vi "Locate Colored Object.vi"() -> ()   [LabVIEW 2013]
doc: "<B>Locate Colored Object</B> searches for objects of a color you select. There are three modes in this program. The first is \"Simple\" that lets you select red, green, or blue, and a sensitivity level. The second is \"Color Wheel\" which allows you to select a hue to search for along a color wheel. The final mode is \"HSL Numbers\" which allows you to set a minimum and maximum for Hue, Saturation, and Luminance. In all three cases a mask display shows any objects that match your parameters as red against a black background."
uses:
  <vilib>/Rock Robotics/WPI/Camera/WPI_CameraFrameRate.ctl
  <vilib>/Rock Robotics/WPI/Camera/WPI_CameraImageSize.ctl
panel:
  in  "Frame Rate (fps)":T1=20 min=1 max=30
  out "Mask":T2(plugin-control)
  out "Rectangle":T3
  in  "Tab Control":enum32{"Simple", "Color Wheel", "HSL Numbers"}(tab)=enum."Color Wheel"
  in  "Sensitivity":dbl(slide) scale=1.0..5.0
  in  "Basic Color":enum32{"Red", "Green", "Blue"}(radio)=enum."Green"
  in  "AutoCal":bool
  in  "Hue Selector":T4={"Hue"=65.11832883917573, "Saturation"=43.78787878787879, "Luminance"=100.45454545454545, "Hue Margin"=20.0} {"Hue Margin" scale=0.0..40.0; "Luminance" scale=0.0..255.0; "Saturation" scale=0.0..255.0; "Hue" scale=0.0..255.0}
  in  "Color Range":T5={"Hue"={"Lower"=55, "Upper"=93}, "Saturation"={"Lower"=73, "Upper"=255}, " Luminance"={"Lower"=99, "Upper"=255}}
  out "fps":dbl=20.0
  out "Particles":i32
  out "Area":i32
  in  "Decimate by":cluster{"H":i32, "V":i32}={"H"=3, "V"=5}
  in  "stop":bool
  # "This example shows a basic object location technique based on color processing.\nIt sets the camera up for medium sized image and passes each images into a subVI\nthat returns the location and size of the largest particle of that color. You can modify the\namount that you decimate the the image to trade speed for precision in location and size.\nThere are three ways to specify the color range.\nThe Simple tab implements a basic autoCalibration, Color wheel uses a center Hue and\nmargin amount, and a saturation and luminance range. The HSL numbers shows the low\nlevel values for complete flexibility."
  # "Determine which color best\ndescribes the target.\n\nMake sure it is in the frame\nand close to the camera,\nthen  press Calibrate.\n\nHigher Sensitivity tightens\nthe fit."
  # "Adjust the color"
  # "You can directly type in HSL threshold numbers.\nThis provides maximum control, but it helps to know\nwhat HSL is. Wikipedia may be able to help with that."
  # "Lower:"
  # "Upper:"
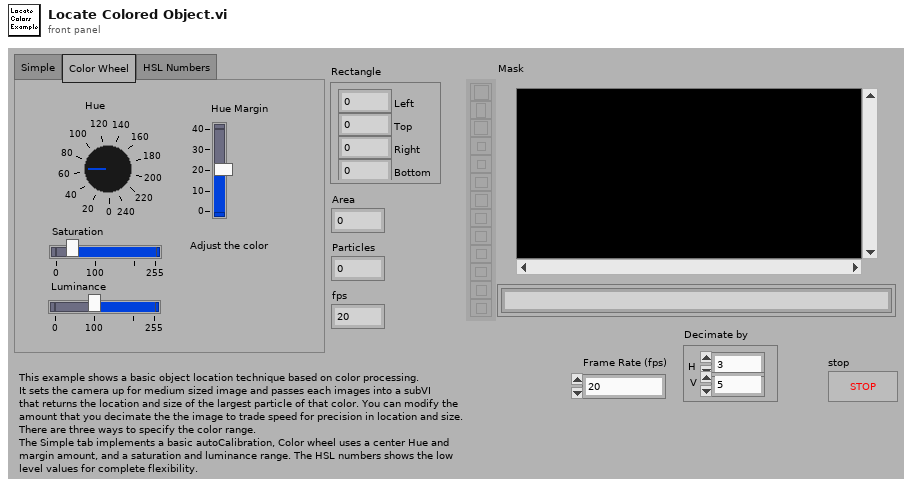
[diagram p1: front panel]
types:
  T1 = typedef "WPI_CameraFrameRate.ctl" = u32
  T2 = typedef "IMAQ Image.ctl" = refnum<image>
  T3 = cluster{"Left":i32, "Top":i32, "Right":i32, "Bottom":i32}
  T4 = cluster{"Hue":dbl, "Saturation":dbl, "Luminance":dbl, "Hue Margin":dbl}
  T5 = cluster{"Hue":cluster{"Lower":u8, "Upper":u8}, "Saturation":cluster{"Lower":u8, "Upper":u8}, " Luminance":cluster{"Lower":u8, "Upper":u8}}
  T6 = typedef "WPI_CameraImageSize.ctl" = enum16{"640x480", "320x240", "160x120"}
  T7 = typedef "Image Type" = u32
  T8 = typedef "WPI_CameraDevRef.ctl" = cluster{"Camera Address":string, "CameraStatus":errorcluster, "Acquire Image Notifier":refnum<notifier>}
  T9 = cluster{cluster{dbl, dbl}, cluster{"Saturation":dbl, i32}, cluster{"Luminance":dbl, i32}}
  T10 = cluster{cluster{sgl, sgl}, cluster{"Mean Value":sgl, "Standard  Deviation":sgl}}
  T11 = cluster{"Mean Value":sgl, "Standard  Deviation":sgl}
  T12 = cluster{cluster{sgl, sgl}, cluster{sgl, sgl}, cluster{sgl, sgl}}
  T13 = cluster{"Mean Value":sgl, sgl, sgl, "Standard  Deviation":sgl}
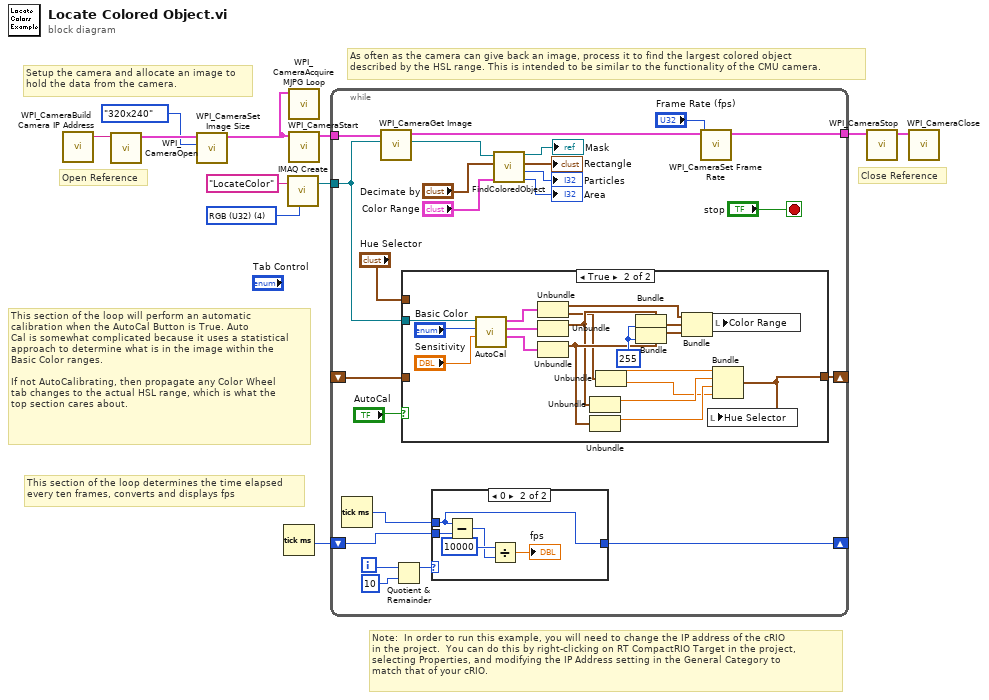
[diagram p0: block diagram]
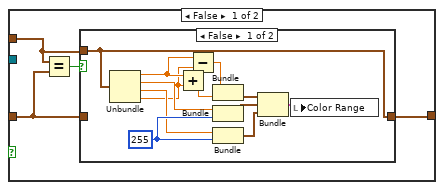
[diagram p2: hidden frame]
diagram:
  w6 = T7 4 items=["Grayscale (U8)", "Grayscale (I16)", "Grayscale (SGL)", "Complex (CSG)", "RGB (U32)", "HSL (U32)", "RGB (U64)", "Grayscale (U16)"] ("Image Type")
  # "Open Reference"
  # "Close Reference"
  # "Note:  In order to run this example, you will need to change the IP address of the cRIO\nin the project.  You can do this by right-clicking on RT CompactRIO Target in the project,\nselecting Properties, and modifying the IP Address setting in the General Category to \nmatch that of your cRIO."
  # "As often as the camera can give back an image, process it to find the largest colored object\ndescribed by the HSL range. This is intended to be similar to the functionality of the CMU camera."
  # "Setup the camera and allocate an image to\nhold the data from the camera."
  # "This section of the loop will perform an automatic\ncalibration when the AutoCal Button is True. Auto\nCal is somewhat complicated because it uses a statistical\napproach to determine what is in the image within the\nBasic Color ranges.\n\nIf not AutoCalibrating, then propagate any Color Wheel\ntab changes to the actual HSL range, which is what the\ntop section cares about."
  # "This section of the loop determines the time elapsed\nevery ten frames, converts and displays fps"
  n1 = call <vilib>:"WPI_CameraBuild Camera IP Address.vi"() -> ("Camera Address"=w2:string)  [unwired: 11 in]
  n2 = call <vilib>:"WPI_CameraOpen.vi"("Camera Address"=w2) -> ("CameraDevRef"=w4:T8)  [unwired: 1 in, 9 out]
  n3 = call <vilib>:"WPI_CameraSet Image Size.vi"("Image Size"=WPI_CameraImageSize."320x240", "CameraDevRef"=w4) -> ("CameraDevRef Out"=w1:T8)  [unwired: 1 in, 8 out]
  n4 = Tick Count (ms)() -> (millisecond timer value=w5:u32)
  n5 = call "IMAQ Create"("Image Name"="LocateColor", "Image Type"=w6) -> ("New Image"=w8:T2)  [unwired: 2 in, 2 out]
  n6 = call <vilib>:"WPI_CameraAcquire MJPG Loop.vi"("CameraDevRef"=w1) -> ()  [unwired: 11 in]
  n7 = call <vilib>:"WPI_CameraStart.vi"("CameraDevRef"=w1) -> ("CameraDevRef Out"=w11:T8)  [unwired: 1 in, 9 out]
  n8 = while {
    tunnel: w11 -> [w33]
    tunnel: [w12] -> w10
    tunnel: w8 -> [w22]
    shift-right: [w24] -> _
    shift-left: w5 -> [w28]
    shift-right: [w16] -> _
    shift-left: _ -> [w17]
    i -> [w26]
    stop <- "stop" stop-if-true
    n9 = Tick Count (ms)() -> (millisecond timer value=w27:u32)
    n10 = call <vilib>:"WPI_CameraGet Image.vi"("Image"=w22, "CameraDevRef"=w33) -> ("Image Out"=w32:T2, "CameraDevRef Out"=w13:T8)  [unwired: 1 in, 7 out]
    n11 = Quotient & Remainder(x=w26, y=10) -> (x-y*floor(x/y)=w25:i32)  [unwired: 1 out]
    n12 = case shown="True" "AutoCal" {
      tunnel: w22 -> [_ w70]
      tunnel: "Hue Selector" -> [w35 _]
      tunnel: w17 -> [w36 _]
      tunnel: [w37 w52] -> w16
      frame False {
        n13 = Equal?(x=w35, y=w36) -> (x = y?=w38:bool)
        n14 = case shown="False" w38 {
          tunnel: w35 -> [w39 _]
          tunnel: [w39 w51] -> w37
          tunnel: w36 -> [_ w51]
          frame False {
            w50 = 255
            n15 = Unbundle(w39) -> ("Hue"=w43:dbl, "Saturation"=w48:dbl, "Luminance"=w49:dbl, "Hue Margin"=w42:dbl)
            n16 = Add(x=w43, y=w42) -> (x+y=w40:dbl)
            n17 = Subtract(x=w43, y=w42) -> (x-y=w41:dbl)
            n18 = Bundle(w41, w40) -> (w45:cluster{dbl, dbl})  [unwired: 1 out]
            n19 = Bundle("Saturation"=w48, w50) -> (w46:cluster{"Saturation":dbl, i32})  [unwired: 1 out]
            n20 = Bundle("Luminance"=w49, w50) -> (w47:cluster{"Luminance":dbl, i32})  [unwired: 1 out]
            n21 = Bundle(w45, w46, w47) -> (w44:T9)  [unwired: 1 out]
            n22 = local write "Color Range"(w44) -> ()
          }
          frame True {
          }
        }
      }
      frame True {
        w60 = 255
        n23 = call "AutoCal.vi"("Std Devs"="Sensitivity", "Target Color"="Basic Color", "Color Image"=w70) -> ("Luminance Info"=w66:T10, "Saturation Info"=w67:T10, "Hue Info"=w69:T10)  [unwired: 6 out]
        n24 = Unbundle(w69) -> (w68:cluster{sgl, sgl}, w55:T11)
        n25 = Unbundle(w67) -> (w57:cluster{sgl, sgl})  [unwired: 1 out]
        n26 = Unbundle(w66) -> (w59:cluster{sgl, sgl})  [unwired: 1 out]
        n27 = Unbundle(w57) -> (w56:sgl)  [unwired: 1 out]
        n28 = Unbundle(w59) -> (w58:sgl)  [unwired: 1 out]
        n29 = Unbundle(w55) -> ("Mean Value"=w53:sgl, "Standard  Deviation"=w54:sgl)
        n30 = Bundle(cluster=w57, w60) -> (w61:cluster{sgl, sgl})  [unwired: 1 out]
        n31 = Bundle(cluster=w59, w60) -> (w62:cluster{sgl, sgl})  [unwired: 1 out]
        n32 = Bundle(w68, w61, w62) -> (w65:T12)  [unwired: 1 out]
        n33 = local write "Color Range"(w65) -> ()
        n34 = Bundle("Mean Value"=w53, w56, w58, "Standard  Deviation"=w54) -> (w52:T13)  [unwired: 1 out]
        n35 = local write "Hue Selector"(w52) -> ()
      }
    }
    n36 = case shown="0" w25 {
      tunnel: w28 -> [w71 w76]
      tunnel: w27 -> [_ w75]
      tunnel: [w71 w75] -> w24
      frame Default {
      }
      frame 0 {
        n37 = Subtract(x=w75, y=w76) -> (x-y=w72:u32)
        n38 = Divide(x=u32 10000 ("y"), y=w72) -> (x/y=→"fps":dbl)
      }
    }
    n39 = call "FindColoredObject.vi"("Color Range"="Color Range", "Decimate by"="Decimate by", "Color Image In"=w32) -> ("Area"=→"Area":i32, "Particles"=→"Particles":i32, "Rectangle"=→"Rectangle":T3, "Mask Image"=→"Mask":T2)  [unwired: 3 out]
    n40 = call <vilib>:"WPI_CameraSet Frame Rate.vi"("Frame Rate (fps)"="Frame Rate (fps)", "CameraDevRef"=w13) -> ("CameraDevRef Out"=w12:T8)  [unwired: 1 in, 8 out]
  }
  n41 = call <vilib>:"WPI_CameraStop.vi"("CameraDevRef"=w10) -> ("CameraDevRef Out"=w9:T8)  [unwired: 1 in, 9 out]
  n42 = call <vilib>:"WPI_CameraClose.vi"("CameraDevRef"=w9) -> ()  [unwired: 1 in, 10 out]
